vi "Generate Report as INI Section.vi"(7 "Parameters":variant, 8 "error in (no error)":errorcluster, 9 "Results":variant, 10 "Refnum in":T1, 11 "Analyze BaseClass in":refnum<class "Analyze BaseClass.lvclass">) -> (0 "error out":errorcluster, 2 "Refnum out":T1, 3 "Analyze BaseClass out":refnum<class "Analyze BaseClass.lvclass">)   [LabVIEW 2020, in "Analyze.lvlib" / "Analyze BaseClass.lvclass"]
uses:
  Analyze BaseClass.lvclass
  <vilib>/Utility/config.llb/Config Data RefNum.ctl
  <vilib>/Utility/config.llb/NI_LVConfig.lvlib
  <vilib>/Utility/config.llb/Write Key (I32).vi
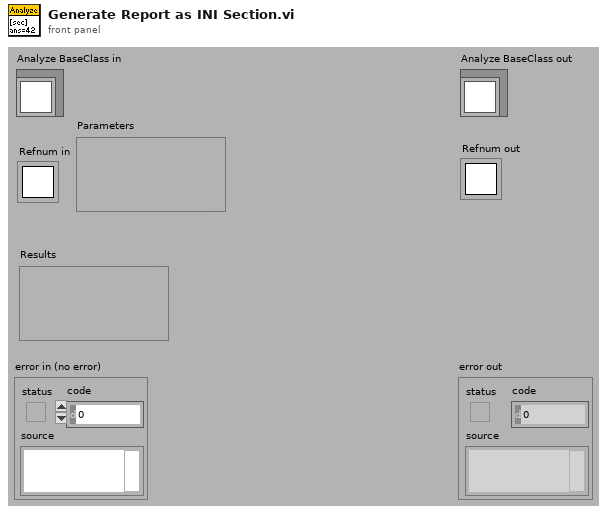
[diagram p1: front panel]
types:
  T1 = typedef "NI_LVConfig.lvlib/Config Data RefNum.ctl" = refnum<k1>
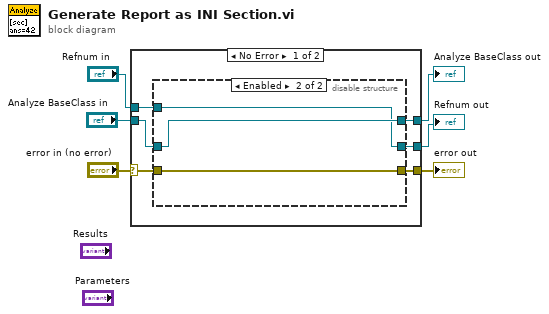
[diagram p0: block diagram]
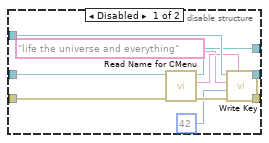
[diagram p2: hidden frame]
diagram:
  n1 = case shown="No Error" "error in (no error)" {
    selector: "error in (no error)" -> [w12 w28]
    tunnel: [w9 w28] -> w5
    tunnel: [w7 w27] -> w3
    tunnel: "Analyze BaseClass in" -> [w8 w27]
    tunnel: [w10 w26] -> w2
    tunnel: "Refnum in" -> [w11 w26]
    frame No Error {
      n2 = disable-structure shown="Enabled" {
        disable-tunnel: w12 -> [w22 w23]
        disable-tunnel: w11 -> [w21 w24]
        disable-tunnel: [w20 w24] -> w10
        disable-tunnel: [w18 w23] -> w9
        disable-tunnel: w8 -> [w17 w25]
        disable-tunnel: [w16 w25] -> w7
        frame Disabled {
          n3 = call-dynamic "Read Name for CMenu.vi"("error in (no error)"=w22, "Analyze BaseClass in"=w17) -> ("error out"=w19:errorcluster, "Name for Context menu"=w15:string, "Analyze BaseClass out"=w16:refnum<class "Analyze BaseClass.lvclass">)  [unwired: 7 in]
          n4 = call-poly <vilib>:"Write Key.vi"("section"=w15, "error in (no error)"=w19, "value"=42, "key"="life the universe and everything", "refnum"=w21) -> ("error out"=w18:errorcluster, "refnum out"=w20:T1)  [unwired: 4 in, 1 out]
        }
        frame Enabled {
        }
      }
    }
    frame Error {
    }
  }
  "error out" <- w5
  "Analyze BaseClass out" <- w3
  "Refnum out" <- w2
